vi "Dashboard Main.vi"() -> ()   [LabVIEW 2015]
uses:
  <vilib>/Utility/miscctls.llb/LVRowAndColumnTypeDef.ctl
  <vilib>/event_ctls.llb/eventvkey.ctl
  <vilib>/Rock Robotics/WPI/Dashboard/WPI_DashboardLogging Global.vi
  <vilib>/Rock Robotics/Network Tables/NT Read Numeric Array.vi
  <vilib>/Utility/config.llb/Write Key (String).vi
  <vilib>/Utility/config.llb/Write Key (I32).vi
  <vilib>/Utility/config.llb/NI_LVConfig.lvlib
panel:
  in  "TCP":refnum<k5>
  in  "Rec Mode":enum32{"Stop", "Record", "Playback"}(radio)
  in  "Vision":u16(ring) items=["Camera Off", "USB Camera SW", "USB Camera HW", "IP Camera"]
  out "Camera IP":string
  out "Image Message":string="Timeout in Camera Communications"
  in  "Dashboard Tab":T1(tab)
  in  "Select Auto":string(combo)
  out "NT Connection":bool
  in  "Camera Settings":T2={"Frame Rate"=30, "Compression"=30, "Size"=1} {"Frame Rate" scale=1.0..30.0; "Size" items=["640x480", "320x240", "160x120"]}
  out "MotorChart R":cluster{"Numeric":dbl, "Numeric":dbl}(graph)
  out "MotorChart L":T3(graph)
  out "MotorSliders R":cluster{"MotorSlide1":dbl, "MotorSlide2":dbl} {"MotorSlide2" scale=-1.0..1.0 scale format="%#_2e"; "MotorSlide1" scale=-1.0..1.0 scale format="%#_2e"}
  out "MotorSliders L":T4 {"MotorSlide4 2" scale=0.0..14.0 scale format="%#_2e"; "MotorSlide2" scale=-1.0..1.0 scale format="%#_2e"; "MotorSlide1" scale=-1.0..1.0 scale format="%#_2e"}
  out "Gyro":dbl(knob) scale=0.0..360.0
  out "JS1 Z":dbl(slide) scale=-1.0..1.0 scale format="%#_2e"
  out "JS1 Graph":cluster{"X":dbl, "Y":dbl}[](graph)
  out "JS1 Buttons":T5
  out "JS2 Z":dbl(slide) scale=-1.0..1.0 scale format="%#_2e"
  out "JS2 Graph":cluster{"X":dbl, "Y":dbl}[](graph)
  out "JS2 Buttons":T5
  out "Mode":T6(ring)=enum."Auto Disabled"
  in  "DB Camera Config":bool
  out "fps":dbl format="%#.1g"
  out "Mbps":dbl format="%#.1g"
  out "Mbps LED":bool
  in  "DB/String 9":string
  in  "DB/String 8":string
  in  "DB/String 7":string
  in  "DB/String 6":string
  in  "DB/String 5":string
  in  "DB/String 4":string
  in  "DB/String 3":string
  in  "DB/String 2":string
  in  "DB/String 1":string
  in  "DB/String 0":string
  in  "DB/Slider 0":dbl(slide) scale=0.0..5.0
  in  "DB/Slider 1":dbl(slide) scale=0.0..5.0
  in  "DB/Slider 2":dbl(slide) scale=0.0..5.0
  in  "DB/Slider 3":dbl(slide) scale=0.0..5.0
  out "DB/LED 3":bool
  out "DB/LED 2":bool
  out "DB/LED 1":bool
  out "DB/LED 0":bool
  in  "DB/Button 3":bool
  in  "DB/Button 2":bool
  in  "DB/Button 1":bool
  in  "DB/Button 0":bool caption="New Name"
  out "Velocity":dbl(knob) scale=0.0..10.0
  in  "Test Slider":dbl(slide) scale=0.0..100.0 scale format="%#_3g"
  in  "On/Off":bool caption="Solenoid"
  in  "Test Name":u16(ring) items=["Select the test to run..."]
  in  "Test Tree":string(tree)
  in  "Motor":cluster{"Value":dbl, "Enable":bool} {"Value" scale=-1.0..1.0 scale format="%#_3g"}
  out "Progress":T7 {"Test Progress" scale=0.0..100.0}
  in  "Rev/Fwd":cluster{"Forward":bool, "Reverse":bool}
  in  "Test Ring":u16(ring) items=["Monochrome", "Color"]
  out "Cmd Status":string
  in  "Execute Command":bool
  in  "Command Params":string[][](table)
  in  "Command Selection":i32(listbox)
  in  "CheckList":i32(listbox)
  out "Tree":string(tree)
  out "Camera Image":T8(plugin-control)
  out "Background":bool
  # "Left"
  # "Front"
  # "Right"
  # "Battery"
  # "This tab is a great place for autonomous settings and robot-specific values.\nPlace controls and indicators inside this tab and match name to\nDashboard Variables on robot. You can also delete this comment."
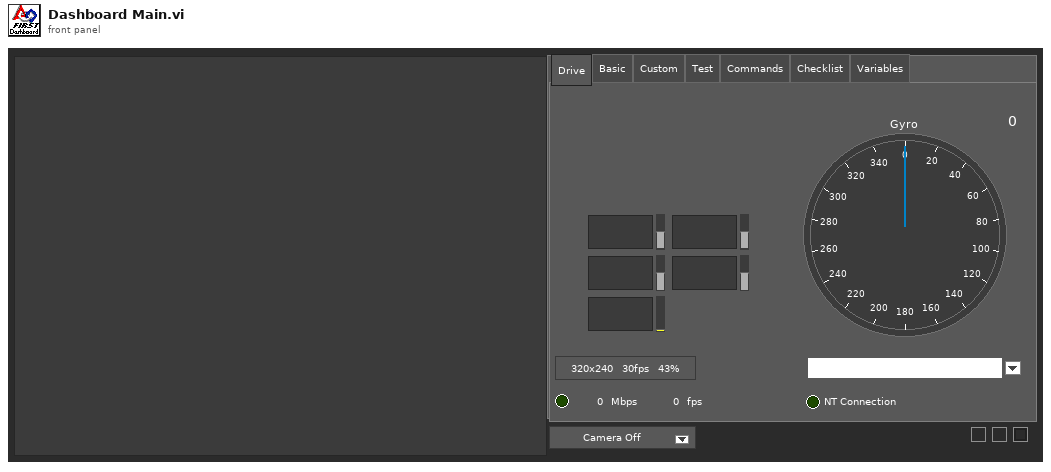
[diagram p1: front panel]
types:
  T1 = enum32{"Drive", "Basic", "Custom", "Test", "Commands", "Checklist", "Variables"}
  T2 = cluster{"Frame Rate":i32, "Compression":i32, "Size":u16}
  T3 = cluster{"Numeric":dbl, "Numeric":dbl, "Battery V":dbl}
  T4 = cluster{"MotorSlide1":dbl, "MotorSlide2":dbl, "MotorSlide4 2":dbl}
  T5 = cluster{bool, bool, bool, bool, bool, bool, bool, bool, bool, bool, bool, bool}
  T6 = enum8{"Tele-Op Disabled", "Tele-Op Enabled", "Auto Disabled", "Auto Enabled", "Test Disabled", "Test Enabled", "Disconnected", "No Code", "E-Stop"}
  T7 = cluster{"Test Progress":u8, "Test Progress Text":string}
  T8 = typedef "IMAQ Image.ctl" = refnum<image>
  T9 = cluster{"IDs":cluster{"RPC field ID":u16, "Unique ID":u16}, "String":string}
  T10 = enum32{"Drive", "Basic", "Custom", "Test", "Checklist", "Variables"}
  T11 = typedef "Image Type" = u32
  T12 = cluster{"Camera Image":refnum<vi>, "Dashboard Tab":refnum<vi>, "Background":refnum<vi>, "Vision":refnum<vi>, "Rec Mode":refnum<vi>, "Test Slider":refnum<vi>, "On/Off ":refnum<vi>, "Test Ring":refnum<vi>, "Rev/Fwd":refnum<vi>, "Test Name":refnum<vi>, "Motor":refnum<vi>, "Progress":refnum<vi>, "CheckList":refnum<vi>, "Tree":refnum<vi>, "Test Tree":refnum<vi>, "Command Params":refnum<vi>, "Command Selection":refnum<vi>, "Execute Command":refnum<vi>, "Cmd Status":refnum<vi>}
  T13 = cluster{"Error Strings":string, "Disable Counts":cluster{u16, u16}, "Rail Faults":cluster{u16, u16, u16}, "Robot IP":string, "DB Mode":u8, "Event Info":cluster{"Name":string, "Type":u8, "Number":u16, "Replay":u8}, "Camera Addr":string}
  T14 = cluster{"Storage":cluster{"Disk Free":u64, "RAM Block":u32, "RAM free":u32}, "CPU Utilization":cluster{"CPU % ISR":sgl, "CPU % Time Crit":sgl, "CPU % Timed Str":sgl, "CPU % High":sgl, "CPU % Above":sgl, "CPU % Normal":sgl, "CPU % Low":sgl}, "CAN":cluster{"% Bus Utilization":sgl, "Bus Off Cnt":u32, "TX_FIFO Full Cnt":u32, "Receive Error Cnt":u8, "Transmit Error Cnt":u8}, "HID":cluster{"HID Outputs":u32, "Rumble Low":u16, "Rumble High":u16}[]}
  T15 = cluster{"Status bits":cluster{"Test Mode":bool, "Autonomous":bool, "Enabled":bool, "Code Start":bool, "Brownout":bool, "Reserved 2":bool, "Reserved 3":bool, "E-Stop":bool}, "Code Trace":cluster{"Disabled":bool, "TeleOp":bool, "Auto":bool, "Test":bool}, "Controller Type":enum16{"unknown", "cRIO", "roboRio"}, "Code?":enum16{"unknown", "noCode", "code"}, "Battery V":dbl}
  T16 = cluster{"Control Bits":cluster{"TestMode":bool, "Autonomous":bool, "Enabled":bool, "FMS Present":bool, bool, bool, bool, "E-Stop":bool}, "Team Station ":u8, "Countdown":sgl, "Joystick Values":cluster{"Axes":dbl[], "Buttons":bool[], "POVs":i16[]}[]}
  T17 = cluster{"Axes":dbl[], "Buttons":bool[], "POVs":i16[]}[]
  T18 = cluster{"Axes":dbl[], "Buttons":bool[], "POVs":i16[]}
  T19 = cluster{"Buttons[0]":bool, "Buttons[1]":bool, "Buttons[2]":bool, "Buttons[3]":bool, "Buttons[4]":bool, "Buttons[5]":bool, "Buttons[6]":bool, "Buttons[7]":bool, "Buttons[8]":bool, "Buttons[9]":bool, "Buttons[10]":bool, "Buttons[11]":bool}
  T20 = typedef "NI_LVConfig.lvlib/Config Data RefNum.ctl" = refnum<k1>
  T21 = cluster{"Operation":enum16{"Update", "Clear"}, "Color Box":u32}[]
  T22 = typedef "eventvkey.ctl" = enum16{"ASCII", "Enter", "Return", "Shift", "Ctrl", "Alt", "Cmd", "Opt", "Caps", "NumLock", "Clear", "Break", "Up", "Down", "Left", "Right", "Insert", "Delete", "Home", "End", "PageUp", "PageDown", "Escape", "Help", "Pause", "ScrollLock", "F1", "F2", "F3", "F4", "F5", "F6", "F7", "F8", "F9", "F10", "F11", "F12", "F13", "F14", "F15", "F16", "F17", "F18", "F19", "F20", "F21", "F22", "F23", "F24", "Play", "VolumeUp", "VolumeDown", "Mute", "Two Byte Char"}
  T23 = cluster{"Image Size":bool, "Image Type":bool, "Pixel Value":bool, "ROI Information":bool, "Zoom Factor":bool}
  T24 = enum8{"Enabled", "Disabled", "Disabled and Grayed Out"}
  T25 = cluster{"Operation":enum16{"Update", "Clear"}, "Color Box":u32}
  T26 = typedef "LVRowAndColumnTypeDef.ctl" = cluster{"Row":i32, "Column":i32}
  T27 = cluster{"Shift":bool, "Ctrl":bool, "Alt":bool, "Cmd":bool, "Opt":bool}
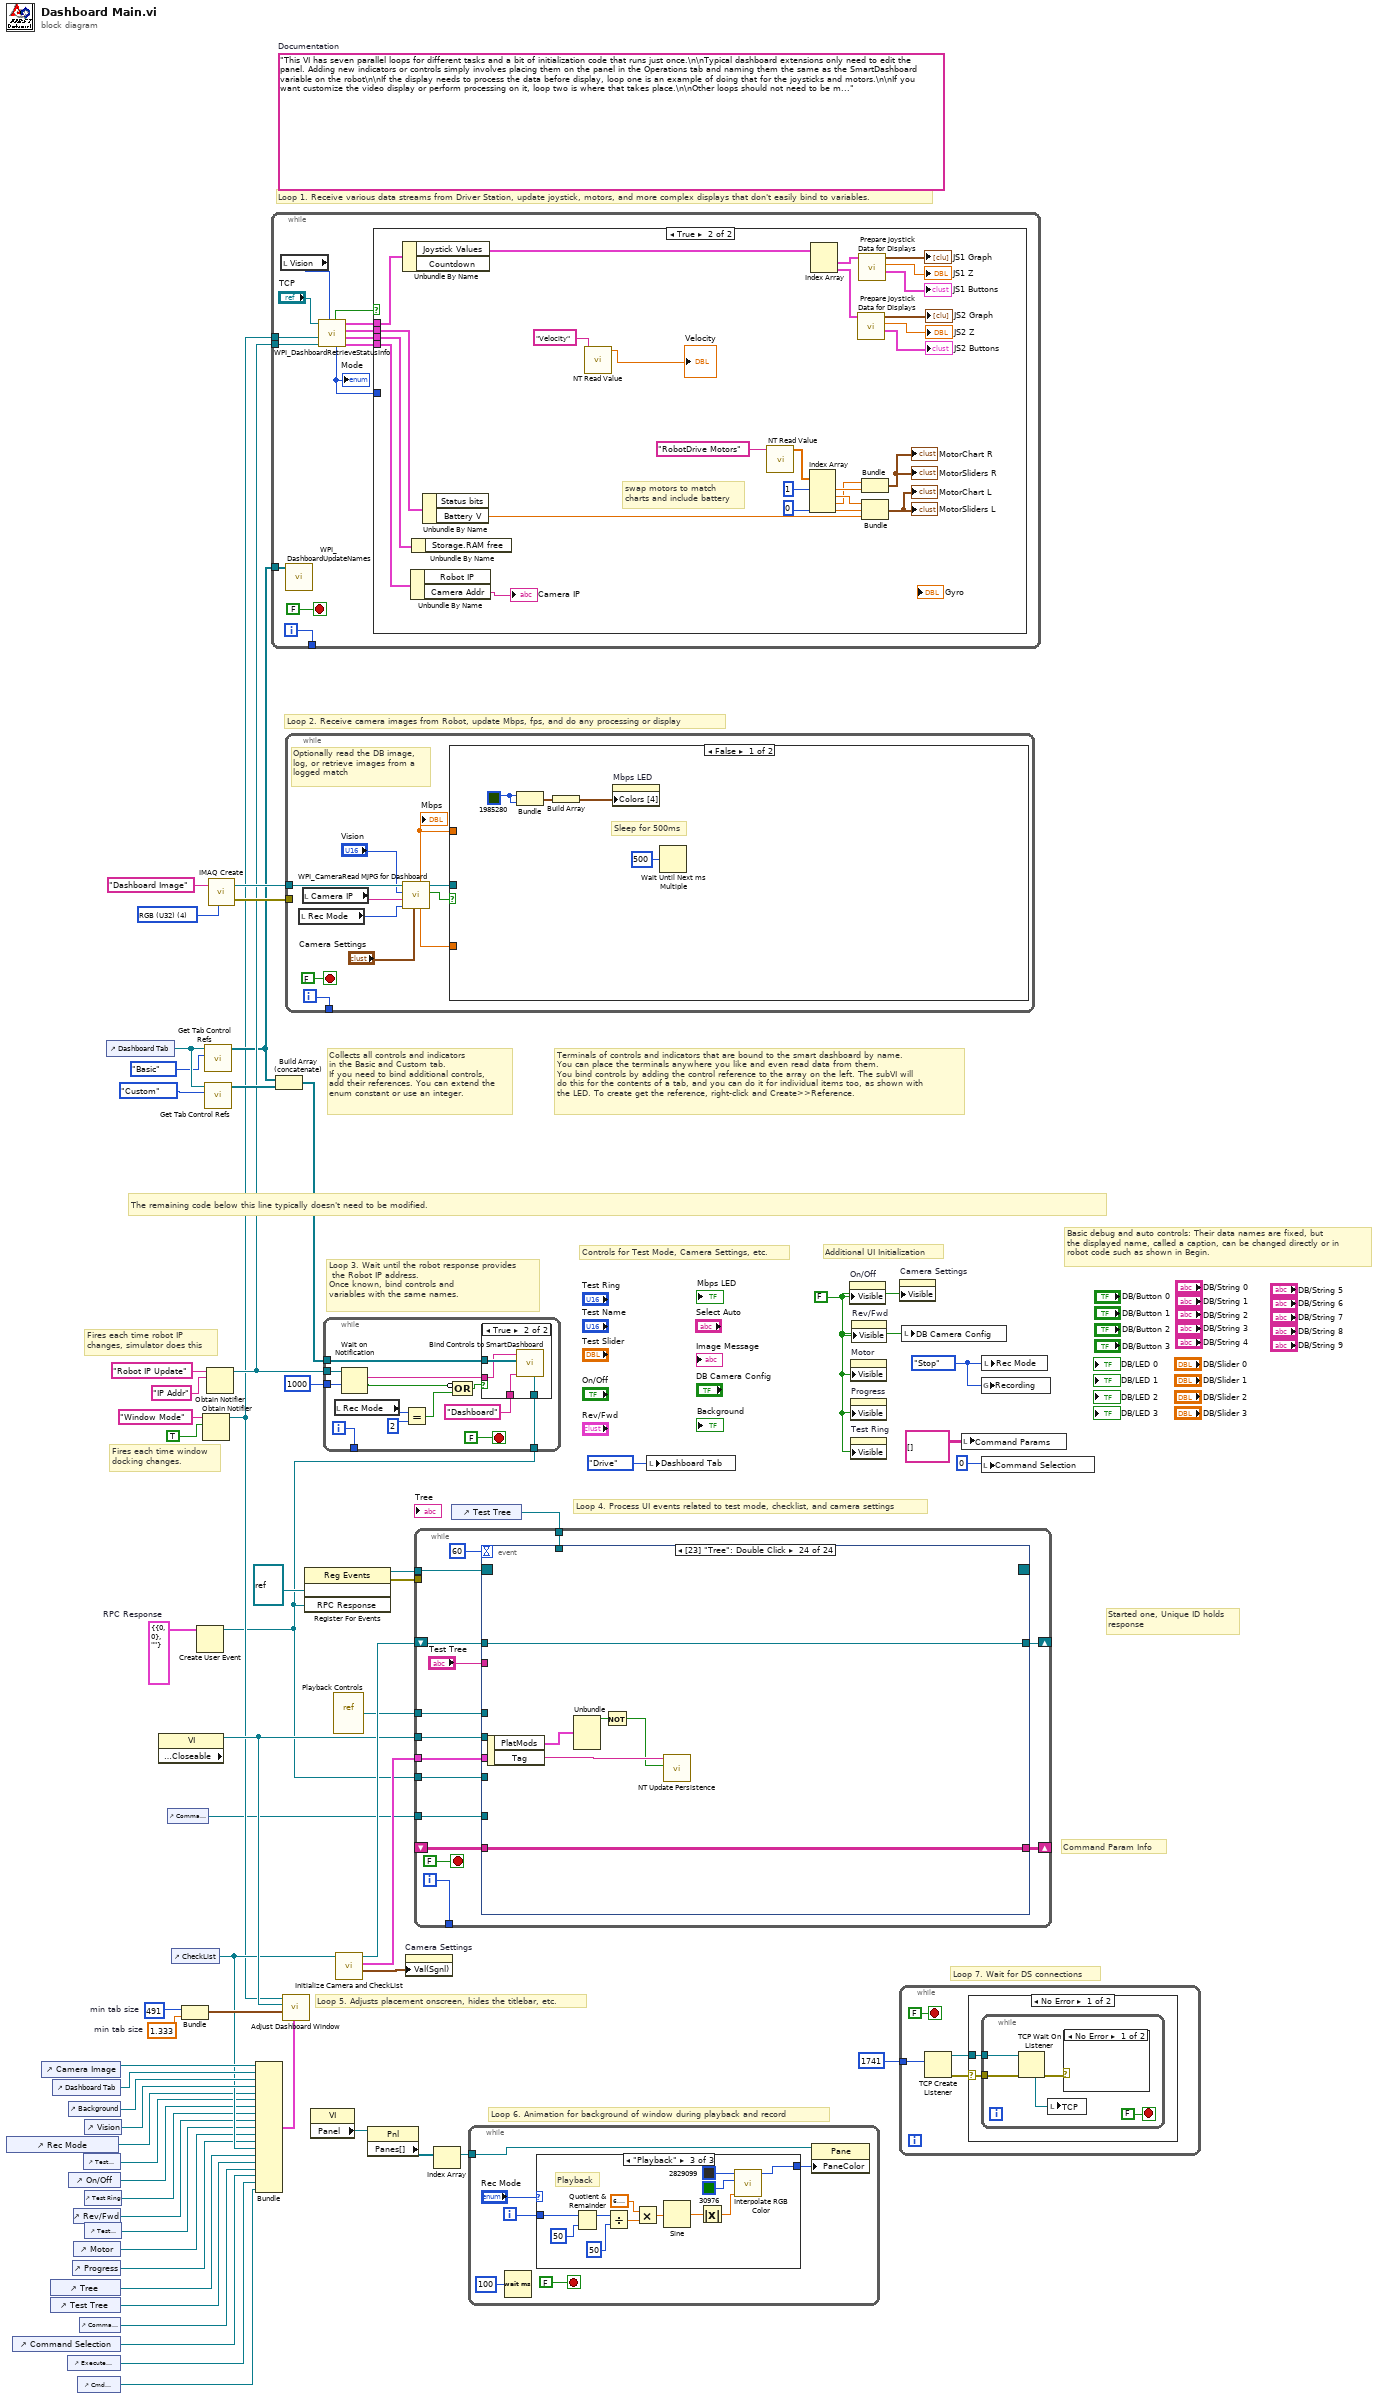
[diagram p0: block diagram]
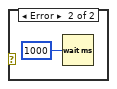
[diagram p2: hidden frame]
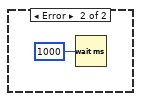
[diagram p3: hidden frame]
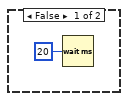
[diagram p4: hidden frame]
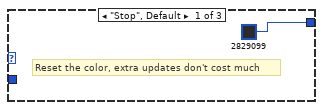
[diagram p5: hidden frame]
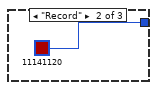
[diagram p6: hidden frame]
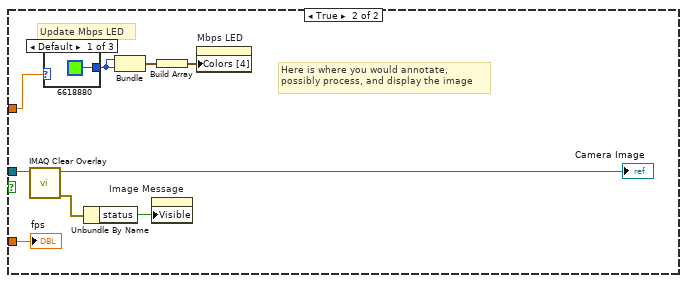
[diagram p8: hidden frame]
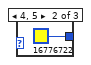
[diagram p9: hidden frame]
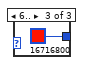
[diagram p10: hidden frame]
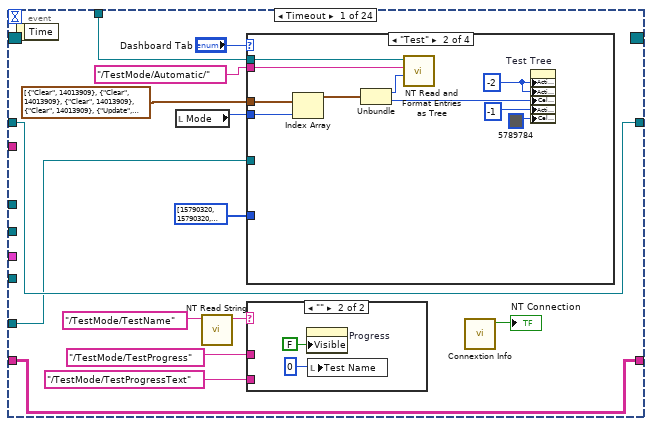
[diagram p11: hidden frame]
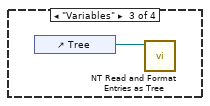
[diagram p13: hidden frame]
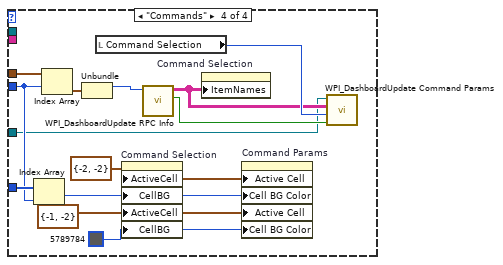
[diagram p14: hidden frame]
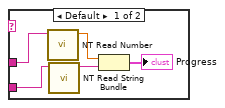
[diagram p15: hidden frame]
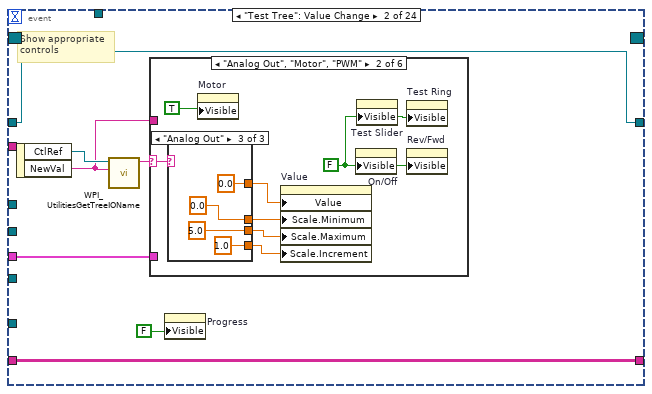
[diagram p16: hidden frame]
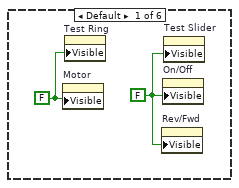
[diagram p17: hidden frame]
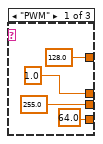
[diagram p18: hidden frame]
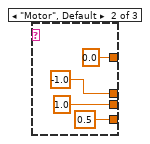
[diagram p19: hidden frame]
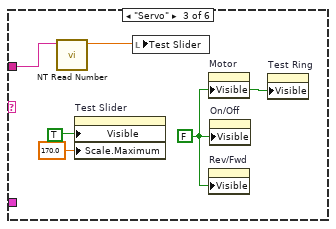
[diagram p20: hidden frame]
diagram:
  w7 = T9 {"IDs"={"RPC field ID"=0, "Unique ID"=0}, "String"=""}  # RPC Response
  w33 = 491  # min tab size
  w32 = 1.333  # min tab size
  w41 = enum32{"Stop", "Record", "Playback"}."Stop" ("Rec Mode")
  w15 = FALSE ("Visible")
  (unwired) "This VI has seven parallel loops for different tasks and a bit of initialization code that runs just once.\n\nTypical dashboard extensions only need to edit the panel. Adding new indicators or controls simply involves placing them on the panel in the Operations tab and naming them the same as the SmartDashboard variable on the robot\n\nIf the display needs to process the data before display, loop one is an example of doing that for the joysticks and motors.\n\nIf you want customize the video display or perform processing on it, loop two is where that takes place.\n\nOther loops should not need to be modified. They are pretty standard, and document the task they perform."  # Documentation
  w61 = T11 4 items=["Grayscale (U8)", "Grayscale (I16)", "Grayscale (SGL)", "Complex (CSG)", "RGB (U32)", "HSL (U32)", "RGB (U64)"] ("Image Type")
  # "Command Param Info"
  # "Started one, Unique ID holds\nresponse"
  # "Loop 7. Wait for DS connections"
  # "Basic debug and auto controls: Their data names are fixed, but\nthe displayed name, called a caption, can be changed directly or in\nrobot code such as shown in Begin."
  # "Controls for Test Mode, Camera Settings, etc."
  # "Additional UI Initialization"
  # "Loop 6. Animation for background of window during playback and record"
  # "Fires each time robot IP\nchanges, simulator does this"
  # "Fires each time window\ndocking changes."
  # "Collects all controls and indicators\nin the Basic and Custom tab.\nIf you need to bind additional controls,\nadd their references. You can extend the\nenum constant or use an integer."
  # "The remaining code below this line typically doesn't need to be modified."
  # "Loop 4. Process UI events related to test mode, checklist, and camera settings"
  # "Terminals of controls and indicators that are bound to the smart dashboard by name.\nYou can place the terminals anywhere you like and even read data from them.\nYou bind controls by adding the control reference to the array on the left. The subVI will\ndo this for the contents of a tab, and you can do it for individual items too, as shown with\nthe LED. To create get the reference, right-click and Create>>Reference."
  # "Loop 3. Wait until the robot response provides\n the Robot IP address.\nOnce known, bind controls and\nvariables with the same names."
  # "Loop 5. Adjusts placement onscreen, hides the titlebar, etc."
  # "Loop 1. Receive various data streams from Driver Station, update joystick, motors, and more complex displays that don't easily bind to variables."
  # "Loop 2. Receive camera images from Robot, update Mbps, fps, and do any processing or display"
  n1 = control-ref of="Rec Mode"() -> (w21:refnum<vi>)
  n2 = control-ref of="Command Selection"() -> (w6:refnum<vi>)
  n3 = control-ref of="Camera Image"() -> (w36:refnum<vi>)
  n4 = control-ref of="Tree"() -> (w25:refnum<vi>)
  n5 = control-ref of="Test Tree"() -> (w24:refnum<vi>)
  n6 = control-ref of="Dashboard Tab"() -> (w35:refnum<vi>)
  n7 = control-ref of="Execute Command"() -> (w8:refnum<vi>)
  n8 = control-ref of="Background"() -> (w30:refnum<vi>)
  n9 = control-ref of="On/Off"() -> (w19:refnum<vi>)
  n10 = control-ref of="Progress"() -> (w16:refnum<vi>)
  n11 = control-ref of="Rev/Fwd"() -> (w17:refnum<vi>)
  n12 = control-ref of="Motor"() -> (w22:refnum<vi>)
  n13 = control-ref of="Cmd Status"() -> (w2:refnum<vi>)
  n14 = control-ref of="Command Params"() -> (w9:refnum<vi>)
  n15 = control-ref of="Test Slider"() -> (w20:refnum<vi>)
  n16 = control-ref of="Vision"() -> (w34:refnum<vi>)
  n17 = control-ref of="Test Ring"() -> (w18:refnum<vi>)
  n18 = control-ref of="Test Name"() -> (w23:refnum<vi>)
  n19 = control-ref of="Dashboard Tab"() -> (w39:refnum<vi>)
  n20 = property class="VI" props=["Front Panel.Closeable"]() -> (reference out=w40:refnum<vi>)  [unwired: 2 in, 2 out]
  n21 = control-ref of="Command Params"() -> (w1:refnum<vi>)
  n22 = control-ref of="CheckList"() -> (w26:refnum<vi>)
  n23 = Bundle("min tab size"=w33, "min tab size"=w32) -> (w31:cluster{"min tab size":i32, "min tab size":dbl})  [unwired: 1 in]
  n24 = Create User Event(user event datatype=w7) -> (user event=w3:refnum<user-event>)  [unwired: 1 in, 1 out]
  n25 = Obtain Notifier(name (unnamed)="Window Mode", notification data type=TRUE) -> (notifier out=w12:refnum<notifier>)  [unwired: 2 in, 2 out]
  n26 = call <vilib>:"Get Tab Control Refs.vi"("Page Index"=T10."Basic" ("Dashboard Tab"), "TabControl in"=w39) -> ("ControlsOnPage"=w13:refnum<vi>[])  [unwired: 9 in]
  n27 = call <vilib>:"Get Tab Control Refs.vi"("Page Index"=T10."Custom" ("Dashboard Tab"), "TabControl in"=w39) -> ("ControlsOnPage"=w38:refnum<vi>[])  [unwired: 9 in]
  n28 = Obtain Notifier(name (unnamed)="Robot IP Update", notification data type="IP Addr" ("name (unnamed)")) -> (notifier out=w14:refnum<notifier>)  [unwired: 2 in, 2 out]
  n29 = call "IMAQ Create"("Image Name"="Dashboard Image", "Image Type"=w61) -> ("New Image"=w59:T8, "error out"=w58:errorcluster)  [unwired: 2 in, 1 out]
  n30 = Bundle("Camera Image"=w36, "Dashboard Tab"=w35, "Background"=w30, "Vision"=w34, "Rec Mode"=w21, "Test Slider"=w20, "On/Off"=w19, "Test Ring"=w18, "Rev/Fwd"=w17, "Test Name"=w23, "Motor"=w22, "Progress"=w16, "CheckList"=w26, "Tree"=w25, "Test Tree"=w24, "Command Params"=w9, "Command Selection"=w6, "Execute Command"=w8, "Cmd Status"=w2) -> (w27:T12)  [unwired: 1 in]
  n31 = while {
    tunnel: [w73] -> _
    tunnel: w14 -> [w67]
    tunnel: w13 -> [w66]
    tunnel: w12 -> [w62]
    i -> [w73]
    stop <- FALSE stop-if-true
    n32 = local read "Vision"() -> (w64:u16)
    n33 = call <vilib>:"WPI_DashboardUpdateNames.vi"("Controls on Tab"=w66) -> ()  [unwired: 11 in]
    n34 = call <vilib>:"WPI_DashboardRetrieveStatusInfo.vi"("Vision"=w64, "Binding Refnum"=w67, "Window Mode Notifier"=w62, "TCP Cnx"="TCP") -> ("Power and Errors"=w68:T13, "Robot Metrics"=w71:T14, "Status Info"=w72:T15, "Control Info"=w69:T16, "Robot Mode"=w65:T6, "Process?"=w70:bool)  [unwired: 2 in]
    "Mode" <- w65
    n35 = case shown="True" w70 {
      tunnel: w72 -> [_ w102]
      tunnel: w71 -> [_ w101]
      tunnel: w69 -> [_ w100]
      tunnel: w68 -> [_ w99]
      tunnel: w65 -> [_ _]
      frame False {
        n36 = Wait (ms)(milliseconds to wait=u32 20) -> ()  [unwired: 1 out]
      }
      frame True {
        # "swap motors to match\ncharts and include battery"
        n37 = Unbundle By Name(w100) -> ("Joystick Values"=w89:T17)  [unwired: 1 out]
        n38 = Unbundle By Name(w99) -> ("Camera Addr"=→"Camera IP":string)  [unwired: 1 out]
        n39 = Unbundle By Name(w101) -> ()  [unwired: 1 out]
        n40 = Unbundle By Name(w102) -> ("Battery V"=w90:dbl)  [unwired: 1 out]
        n41 = call-poly <vilib>:"NT Read Value.vi"("Name"="Velocity") -> ("Numeric"=→"Velocity":dbl)  [unwired: 9 in, 1 out]
        n42 = call-poly <vilib>:"NT Read Value.vi"("Name"="RobotDrive Motors") -> ("Numeric Array"=w78:dbl[])  [unwired: 9 in, 1 out]
        n43 = Index Array(array=w78, index #1=1, index #4=0) -> (element #1=w94:dbl, element #2=w95:dbl, element #3=w93:dbl, element #4=w98:dbl)  [unwired: 2 in]
        n44 = Index Array(array=w89) -> (element #1=w88:T18, element #2=w83:T18)  [unwired: 2 in]
        n45 = call "Prepare Joystick Data for Displays.vi"("Joystick Values"=w83) -> ("Buttons"=→"JS2 Buttons":T19, "Z Axis"=→"JS2 Z":dbl, "Cartesian Data"=→"JS2 Graph":cluster{"X axis":dbl, "X axis":dbl}[])  [unwired: 8 in]
        n46 = call "Prepare Joystick Data for Displays.vi"("Joystick Values"=w88) -> ("Buttons"=→"JS1 Buttons":T19, "Z Axis"=→"JS1 Z":dbl, "Cartesian Data"=→"JS1 Graph":cluster{"X axis":dbl, "X axis":dbl}[])  [unwired: 8 in]
        n47 = Bundle("Numeric"=w93, "Numeric"=w94) -> (→"MotorChart R" →"MotorSliders R":cluster{"Numeric":dbl, "Numeric":dbl})  [unwired: 1 in]
        n48 = Bundle("Numeric"=w95, "Numeric"=w98, "Battery V"=w90) -> (→"MotorChart L" →"MotorSliders L":T3)  [unwired: 1 in]
      }
    }
  }
  n49 = Build Array (concatenate)(w13, w38) -> (w37:refnum<vi>[])
  n50 = call "Adjust Dashboard Window.vi"("Sizing Refnums"=w27, "Size Constraints"=w31, "VI"=w40, "WIn Mode"=w12) -> ()  [unwired: 8 in]
  n51 = while {
    tunnel: w59 -> [w111]
    tunnel: w58 -> [_]
    tunnel: [w112] -> _
    i -> [w112]
    stop <- FALSE stop-if-true
    # "Optionally read the DB image,\nlog, or retrieve images from a\nlogged match"
    n52 = local read "Rec Mode"() -> (w106:enum32{"Stop", "Record", "Playback"})
    n53 = local read "Camera IP"() -> (w104:string)
    n54 = call <vilib>:"WPI_CameraRead MJPG for Dashboard.vi"("Camera Settings"="Camera Settings", "Rec Mode"=w106, "Camera IP"=w104, "Camera Mode"="Vision", "Refnum in"=w111) -> ("Active"=w109:bool, "Refnum out"=w110:T8, "FPS"=w108:dbl, "Bandwidth (Mbps)"=w103:dbl)  [unwired: 3 in]
    "Mbps" <- w103
    n55 = case shown="False" w109 {
      tunnel: w110 -> [_ w121]
      tunnel: w103 -> [_ w120]
      tunnel: w108 -> [_ w118]
      frame False {
        w114 = u32 1985280 ("Color Box")
        # "Sleep for 500ms"
        n56 = Bundle("Color Box"=w114, "Color Box"=w114) -> (w116:cluster{"Color Box":u32, "Color Box":u32})  [unwired: 1 out]
        n57 = Build Array(w116) -> (w115:cluster{"Color Box":u32, "Color Box":u32}[])
        n58 = property on="Mbps LED" class="Bool (strict)"("Colors [4]"=w115) -> ()  [unwired: 2 in, 2 out]
        n59 = Wait Until Next ms Multiple(millisecond multiple=u32 500) -> ()  [unwired: 1 out]
      }
      frame True {
        # "Here is where you would annotate,\npossibly process, and display the image"
        # "Update Mbps LED"
        n60 = call "IMAQ Clear Overlay"("Image"=w121) -> ("error out"=w125:errorcluster, "Image Out"=→"Camera Image":T8)  [unwired: 2 in, 7 out]
        n61 = case shown="Default" w120 {
          tunnel: [u32 6618880 ("Color Box") u32 16776722 ("Color Box") u32 16716800 ("Color Box")] -> w122
          frame Default {
          }
          frame 4, 5 {
          }
          frame 6.. {
          }
        }
        n62 = Unbundle By Name(w125) -> ("status"=w126:bool)
        n63 = Bundle("Color Box"=w122, "Color Box"=w122) -> (w124:cluster{"Color Box":u32, "Color Box":u32})  [unwired: 1 out]
        n64 = property on="Image Message" class="Str"("Visible"=w126) -> ()  [unwired: 2 in, 2 out]
        n65 = Build Array(w124) -> (w123:cluster{"Color Box":u32, "Color Box":u32}[])
        n66 = property on="Mbps LED" class="Bool (strict)"("Colors [4]"=w123) -> ()  [unwired: 2 in, 2 out]
        "fps" <- w118
      }
    }
  }
  n67 = register-events(refnum<vi> refnum, w3) -> (reference out=w45:refnum<event-registration>, error out=w44:errorcluster)  [unwired: 2 in]
  n68 = property class="VI"() -> ("Panel"=w48:refnum<vi>)  [unwired: 2 in, 2 out]
  n69 = while {
    tunnel: w37 -> [w142]
    tunnel: w14 -> [w140]
    tunnel: [w138] -> _
    tunnel: u32 1000 ("milliseconds to wait") -> [w137]
    tunnel: w3 -> [w130]
    i -> [w138]
    stop <- FALSE stop-if-true
    n70 = local read "Rec Mode"() -> (w133:enum32{"Stop", "Record", "Playback"})
    n71 = Wait on Notification(notifier=w140, timeout in ms (-1)=w137) -> (notification=w139:string, timed out?=w135:bool)  [unwired: 2 in, 2 out]
    n72 = Equal?(x=w133, y=u16 2 ("Rec Mode")) -> (x = y?=w134:bool)
    n73 = Compound Arithmetic op=OR(invert w135, w134) -> (w136:bool)
    n74 = case shown="True" w136 {
      tunnel: w142 -> [_ w146]
      tunnel: w139 -> [_ w145]
      tunnel: "Dashboard" -> [_ w144]
      tunnel: w130 -> [_ w143]
      frame False {
      }
      frame True {
        n75 = call <vilib>:"Bind Controls to SmartDashboard.vi"("RPC ref"=w143, "Client Name"=w144, "Bound Control Refs"=w146, "Server IP Address"=w145) -> ()  [unwired: 8 in]
      }
    }
  }
  n76 = vi-ref "Playback Controls.vi"() -> (w46:refnum<vi>)
  n77 = call "Initialize Camera and CheckList.vi"("ListBox in"=w26) -> ("Cluster"=w52:cluster{"value":i32, "value":i32, "index":i32}, "Array"=w53:cluster{string[]}[], "File Refnum"=w51:T20)  [unwired: 8 in]
  n78 = property class="Pnl"(reference=w48) -> ("Panes[]"=w49:refnum<vi>[])  [unwired: 1 in, 2 out]
  n79 = property on="Camera Settings" class="Clust (strict)"("Val(Sgnl)"=w52) -> ()  [unwired: 2 in, 2 out]
  n80 = Index Array(array=w49) -> (element=w47:refnum<vi>)  [unwired: 1 in]
  n81 = control-ref of="Test Tree"() -> (w50:refnum<vi>)
  n82 = while {
    tunnel: w53 -> [w158]
    shift-right: [w157] -> _
    shift-left: w51 -> [w156]
    tunnel: [w155] -> _
    tunnel: w50 -> [w154]
    tunnel: w46 -> [w153]
    tunnel: w45 -> [w152]
    tunnel: w44 -> [_]
    tunnel: w40 -> [w151]
    tunnel: w3 -> [w150]
    tunnel: w1 -> [w149]
    shift-right: [w148] -> _
    shift-left: _ -> [w147]
    i -> [w155]
    stop <- FALSE stop-if-true
    n83 = event shown="[23] \"Tree\": Double Click" {
      selector: w152 -> [_ _ _ _ _ _ _ _ _ _ _ _ _ _ _ _ _ _ _ _ _ _ _ _]
      dyn-events: [_ _ _ _ _ _ _ _ _ _ _ _ _ _ _ _ _ _ w467 _ _ _ _ _] -> _
      timeout: u32 60 ("milliseconds to wait") -> [_ _ _ _ _ _ _ _ _ _ _ _ _ _ _ _ _ _ _ _ _ _ _ _]
      tunnel: w154 -> [w171 _ _ _ _ _ _ _ _ _ _ _ _ _ _ _ _ _ _ _ _ _ _ _]
      tunnel: "Test Tree" -> [_ _ _ _ _ _ _ _ _ _ _ _ _ w430 w439 w442 w447 w456 _ _ _ _ _ _]
      tunnel: w158 -> [_ w209 _ _ _ _ _ _ _ _ _ w392 w423 _ _ _ _ _ _ _ _ _ _ _]
      tunnel: [w168 w208 w312 w318 w328 w332 w338 w350 w358 w364 w377 w391 w416 w429 w437 w441 w446 w455 w469 w485 w487 w495 w506 w511] -> w157
      tunnel: w156 -> [w168 w208 w312 w318 w328 w332 w338 w350 w358 w364 w377 w390 w416 w429 w437 w441 w446 w455 w469 w485 w487 w495 w506 w511]
      tunnel: w153 -> [_ _ _ _ _ _ _ _ _ _ _ _ _ _ _ _ _ _ w470 _ w490 _ _ _]
      tunnel: w151 -> [_ _ _ _ _ _ _ _ _ _ _ _ _ _ _ _ _ _ w465 _ _ _ _ _]
      tunnel: w150 -> [_ _ _ _ _ _ _ _ _ _ _ _ _ _ _ _ _ _ w461 _ _ _ _ _]
      tunnel: w149 -> [w163 _ _ _ _ _ w336 _ _ _ _ _ _ _ _ _ _ _ _ _ _ _ _ _]
      tunnel: [w162 w207 w311 w317 w327 w333 w334 w344 w355 w363 w376 w389 w415 w428 w436 w440 w445 w454 w460 w483 w486 w491 w499 w512] -> w148
      tunnel: w147 -> [w162 w207 w311 w317 w327 w333 w334 _ _ w363 w376 w389 w415 w428 w436 w440 w445 w454 w460 w483 w486 w491 w499 w512]
      event Timeout {
        n84 = event-data() -> ()  [unwired: 1 in, 1 out]
        n85 = local read "Mode"() -> (w165:T6)
        n86 = call <vilib>:"NT Read String.vi"("Name"="/TestMode/TestName") -> ("String"=w174:string)  [unwired: 9 in, 1 out]
        n87 = case shown="\"Test\"" "Dashboard Tab" {
          tunnel: w171 -> [_ w185 _ _]
          tunnel: "/TestMode/Automatic/" ("Name Pattern") -> [_ w184 _ _]
          tunnel: T21 [{"Operation"=enum."Clear", "Color Box"=14013909}, {"Operation"=enum."Clear", "Color Box"=14013909}, {"Operation"=enum."Clear", "Color Box"=14013909}, {"Operation"=enum."Clear", "Color Box"=14013909}, {"Operation"=enum."Update", "Color Box"=14013909}, {"Operation"=enum."Update", "Color Box"=16777215}, {"Operation"=enum."Clear", "Color Box"=14013909}, {"Operation"=enum."Clear", "Color Box"=14013909}, {"Operation"=enum."Clear", "Color Box"=14013909}] -> [_ w177 _ w194]
          tunnel: w165 -> [_ w176 _ w193]
          tunnel: u32[] [15790320, 15790320, 15790320, 15790320, 16777215, 16777215, 15790320, 15790320, 15790320] -> [_ _ _ w199]
          tunnel: w163 -> [_ _ _ w187]
          frame "Custom", Default {
          }
          frame "Test" {
            w183 = -2 ("Active Item:Row Number")
            n88 = Index Array(array=w177, index=w176) -> (element=w178:T25)
            n89 = Unbundle(w178) -> ("Operation"=w179:enum16{"Update", "Clear"}, "Color Box"=w180:u32)
            n90 = call <vilib>:"NT Read and Format Entries as Tree.vi"("Operation"=w179, "Name Pattern"=w184, "Tree Refnum"=w185) -> ()  [unwired: 7 in, 2 out]
            n91 = property on="Test Tree" class="Tree (strict)"("Active Item Row Number"=w183, "ActiveColNum"=w183, "CellBG"=w180, "Active Item Row Number"=-1 ("Active Item:Row Number"), "CellBG"=u32 5789784 ("Color Box")) -> ()  [unwired: 2 in, 2 out]
          }
          frame "Variables" {
            n92 = control-ref of="Tree"() -> (w186:refnum<vi>)
            n93 = call <vilib>:"NT Read and Format Entries as Tree.vi"("Tree Refnum"=w186) -> ()  [unwired: 9 in, 2 out]
          }
          frame "Commands" {
            w195 = u32 5789784 ("Color Box")
            w196 = T26 {"Row"=-1, "Column"=-2} ("Active Cell:Active Cell")
            w198 = T26 {"Row"=-2, "Column"=-2} ("Active Cell:Active Cell")
            n94 = Index Array(array=w199, index=w193) -> (element=w197:u32)
            n95 = Index Array(array=w194, index=w193) -> (element=w192:T25)
            n96 = Unbundle(w192) -> ("Operation"=w191:enum16{"Update", "Clear"})  [unwired: 1 out]
            n97 = local read "Command Selection"() -> (w190:i32)
            n98 = property on="Command Selection" class="MCListbox (strict)"("ActiveCell"=w198, "CellBG"=w197, "ActiveCell"=w196, "CellBG"=w195) -> ()  [unwired: 2 in, 2 out]
            n99 = call <vilib>:"WPI_DashboardUpdate RPC Info.vi"("Operation"=w191) -> ("update"=w189:bool, "commands"=w188:string[][])  [unwired: 9 in]
            n100 = property on="Command Selection" class="MCListbox (strict)"("ItemNames"=w188) -> ()  [unwired: 2 in, 2 out]
            n101 = property on="Command Params" class="Tbl (strict)"("Active Cell"=w198, "Cell BG Color"=w197, "Active Cell"=w196, "Cell BG Color"=w195) -> ()  [unwired: 2 in, 2 out]
            n102 = call <vilib>:"WPI_DashboardUpdate Command Params.vi"("Update"=w189, "NewVal"=w190, "Commands"=w188, "Param Tbl"=w187) -> ()  [unwired: 7 in, 1 out]
          }
        }
        n103 = case shown="\"\"" w174 {
          tunnel: "/TestMode/TestProgress" ("Name") -> [w201 _]
          tunnel: "/TestMode/TestProgressText" ("Name") -> [w200 _]
          frame Default {
            n104 = call <vilib>:"NT Read Number.vi"("Name"=w201) -> ("Numeric"=w202:dbl)  [unwired: 9 in, 1 out]
            n105 = call <vilib>:"NT Read String.vi"("Name"=w200) -> ("String"=w203:string)  [unwired: 9 in, 1 out]
            n106 = Bundle("Numeric"=w202, "String"=w203) -> (→"Progress":cluster{"Numeric":dbl, "String":string})  [unwired: 1 in]
          }
          frame "" {
            n107 = property on="Progress" class="Clust (strict)"("Visible"=FALSE) -> ()  [unwired: 2 in, 2 out]
            n108 = local write "Test Name"(u16 0) -> ()
          }
        }
        n109 = call <vilib>:"Connextion Info.vi"() -> ("Connected"=→"NT Connection":bool)  [unwired: 10 in, 1 out]
      }
      event "Test Tree": Value Change {
        # "Show appropriate\ncontrols"
        n110 = event-data() -> ("CtlRef"=w212:refnum<vi>, "NewVal"=w210:string)  [unwired: 1 in]
        n111 = call <vilib>:"WPI_UtilitiesGetTreeIOName.vi"("NewVal"=w210, "TreeControl in"=w212) -> ("I/O Name"=w213:string)  [unwired: 9 in]
        n112 = case shown="\"Analog Out\", \"Motor\", \"PWM\"" w213 {
          selector: w213 -> [_ w220 _ w242 w251 _]
          tunnel: w210 -> [_ _ w239 w241 _ w258]
          tunnel: w209 -> [_ _ _ _ _ w257]
          frame Default {
            w215 = FALSE ("Visible")
            w214 = FALSE ("Visible")
            n113 = property on="Motor" class="Clust (strict)"("Visible"=w214) -> ()  [unwired: 2 in, 2 out]
            n114 = property on="Test Ring" class="Ring (strict)"("Visible"=w214) -> ()  [unwired: 2 in, 2 out]
            n115 = property on="Rev/Fwd" class="Clust (strict)"("Visible"=w215) -> ()  [unwired: 2 in, 2 out]
            n116 = property on="On/Off" class="Bool (strict)"("Visible"=w215) -> ()  [unwired: 2 in, 2 out]
            n117 = property on="Test Slider" class="Slide (strict)"("Visible"=w215) -> ()  [unwired: 2 in, 2 out]
          }
          frame "Analog Out", "Motor", "PWM" {
            w221 = FALSE ("Visible")
            n118 = case shown="\"Analog Out\"" w220 {
              tunnel: [1.0 ("Value") -1.0 ("Value") 0.0 ("Value")] -> w219
              tunnel: [255.0 ("Value") 1.0 ("Value") 5.0 ("Value")] -> w218
              tunnel: [128.0 ("Value") 0.0 ("Value") 0.0 ("Value")] -> w217
              tunnel: [64.0 ("Value") 0.5 ("Value") 1.0 ("Value")] -> w216
              frame "PWM" {
              }
              frame "Motor", Default {
              }
              frame "Analog Out" {
              }
            }
            n119 = property on="Motor" class="Clust (strict)"("Visible"=TRUE) -> ()  [unwired: 2 in, 2 out]
            n120 = property on="Value" class="Slide (strict)"("Value"=w217, "Scale.Minimum"=w219, "Scale.Maximum"=w218, "Scale.Increment"=w216) -> ()  [unwired: 2 in, 2 out]
            n121 = property on="On/Off" class="Bool (strict)"("Visible"=w221) -> ()  [unwired: 2 in, 2 out]
            n122 = property on="Test Slider" class="Slide (strict)"("Visible"=w221) -> ()  [unwired: 2 in, 2 out]
            n123 = property on="Test Ring" class="Ring (strict)"("Visible"=w221) -> ()  [unwired: 2 in, 2 out]
            n124 = property on="Rev/Fwd" class="Clust (strict)"("Visible"=w221) -> ()  [unwired: 2 in, 2 out]
          }
          frame "Servo" {
            w237 = FALSE ("Visible")
            n125 = call <vilib>:"NT Read Number.vi"("Name"=w239) -> ("Numeric"=w238:dbl)  [unwired: 9 in, 1 out]
            n126 = property on="Test Slider" class="Slide (strict)"("Visible"=TRUE, "Scale.Maximum"=170.0 ("Scale.Range:Maximum")) -> ()  [unwired: 2 in, 2 out]
            n127 = local write "Test Slider"(w238) -> ()
            n128 = property on="Motor" class="Clust (strict)"("Visible"=w237) -> ()  [unwired: 2 in, 2 out]
            n129 = property on="Rev/Fwd" class="Clust (strict)"("Visible"=w237) -> ()  [unwired: 2 in, 2 out]
            n130 = property on="On/Off" class="Bool (strict)"("Visible"=w237) -> ()  [unwired: 2 in, 2 out]
            n131 = property on="Test Ring" class="Ring (strict)"("Visible"=w237) -> ()  [unwired: 2 in, 2 out]
          }
          frame "Relay", "Solenoid" {
            w240 = FALSE ("Visible")
            n132 = property on="Motor" class="Clust (strict)"("Visible"=w240) -> ()  [unwired: 2 in, 2 out]
            n133 = property on="Test Slider" class="Slide (strict)"("Visible"=w240) -> ()  [unwired: 2 in, 2 out]
            n134 = Search and Replace String(input string=w241, search string="/Value  **", replace string="/Direction") -> (result string=w247:string)  [unwired: 5 in, 3 out]
            n135 = property on="Test Ring" class="Ring (strict)"("Visible"=w240) -> ()  [unwired: 2 in, 2 out]
            n136 = call <vilib>:"NT Read String.vi"("Name"=w247) -> ("String"=w245:string)  [unwired: 9 in, 1 out]
            n137 = Equal?(x="Both directions", y=w245) -> (x = y?=w243:bool)
            n138 = Not(x=w243) -> (.not. x?=w244:bool)
            n139 = property on="Rev/Fwd" class="Clust (strict)"("Visible"=w243) -> ()  [unwired: 2 in, 2 out]
            n140 = property on="On/Off" class="Bool (strict)"("Visible"=w244, "Caption.Text"=w242) -> ()  [unwired: 2 in, 2 out]
          }
          frame "Compressor", "Digital Out" {
            w250 = FALSE ("Visible")
            # "Get direction and finish"
            n141 = property on="Motor" class="Clust (strict)"("Visible"=w250) -> ()  [unwired: 2 in, 2 out]
            n142 = property on="Test Slider" class="Slide (strict)"("Visible"=w250) -> ()  [unwired: 2 in, 2 out]
            n143 = property on="Test Ring" class="Ring (strict)"("Visible"=w250) -> ()  [unwired: 2 in, 2 out]
            n144 = property on="On/Off" class="Bool (strict)"("Visible"=TRUE, "Caption.Text"=w251) -> ()  [unwired: 2 in, 2 out]
            n145 = property on="Rev/Fwd" class="Clust (strict)"("Visible"=FALSE) -> ()  [unwired: 2 in, 2 out]
          }
          frame "Camera" {
            n146 = call <vilib>:"Get Last Path Segment.vi"("String in"=w258) -> ("String out"=w259:string)  [unwired: 10 in]
            n147 = property on="On/Off" class="Bool (strict)"("Visible"=FALSE) -> ()  [unwired: 2 in, 2 out]
            n148 = property on="Motor" class="Clust (strict)"("Visible"=FALSE) -> ()  [unwired: 2 in, 2 out]
            n149 = property on="Rev/Fwd" class="Clust (strict)"("Visible"=FALSE) -> ()  [unwired: 2 in, 2 out]
            n150 = case shown="\"White Balance  **\"" w259 {
              tunnel: w258 -> [w265 w274 w283 w292 w301 _ w307]
              tunnel: w257 -> [w263 w271 w280 w289 w298 _ _]
              frame "Size  **" {
                n151 = Index Array(array=w263) -> (element=w262:cluster{string[]})  [unwired: 1 in]
                n152 = call <vilib>:"NT Read String.vi"("Name"=w265) -> ("String"=w264:string)  [unwired: 9 in, 1 out]
                n153 = Unbundle(w262) -> (w260:string[])
                n154 = Match First String(2:w260, 3:w264) -> (0:w261:i32)  [unwired: 1 out]
                n155 = property on="Test Ring" class="Ring (strict)"("Value"=w261, "Strings []"=w260) -> ()  [unwired: 2 in, 2 out]
                n156 = property on="Test Ring" class="Ring (strict)"("Visible"=TRUE) -> ()  [unwired: 2 in, 2 out]
                n157 = property on="Test Slider" class="Slide (strict)"("Visible"=FALSE) -> ()  [unwired: 2 in, 2 out]
              }
              frame "White Balance  **" {
                n158 = Index Array(array=w271, index=1) -> (element=w272:cluster{string[]})
                n159 = call <vilib>:"NT Read String.vi"("Name"=w274) -> ("String"=w273:string)  [unwired: 9 in, 1 out]
                n160 = Unbundle(w272) -> (w269:string[])
                n161 = Match First String(2:w269, 3:w273) -> (0:w268:i32)  [unwired: 1 out]
                n162 = property on="Test Ring" class="Ring (strict)"("Value"=w268, "Strings []"=w269) -> ()  [unwired: 2 in, 2 out]
                n163 = property on="Test Ring" class="Ring (strict)"("Visible"=TRUE) -> ()  [unwired: 2 in, 2 out]
                n164 = property on="Test Slider" class="Slide (strict)"("Visible"=FALSE) -> ()  [unwired: 2 in, 2 out]
              }
              frame "Exposure  **" {
                n165 = Index Array(array=w280, index=2) -> (element=w281:cluster{string[]})
                n166 = call <vilib>:"NT Read String.vi"("Name"=w283) -> ("String"=w282:string)  [unwired: 9 in, 1 out]
                n167 = Unbundle(w281) -> (w277:string[])
                n168 = Match First String(2:w277, 3:w282) -> (0:w278:i32)  [unwired: 1 out]
                n169 = property on="Test Ring" class="Ring (strict)"("Value"=w278, "Strings []"=w277) -> ()  [unwired: 2 in, 2 out]
                n170 = property on="Test Ring" class="Ring (strict)"("Visible"=TRUE) -> ()  [unwired: 2 in, 2 out]
                n171 = property on="Test Slider" class="Slide (strict)"("Visible"=FALSE) -> ()  [unwired: 2 in, 2 out]
              }
              frame "Exposure Priority  **" {
                n172 = Index Array(array=w289, index=3) -> (element=w290:cluster{string[]})
                n173 = call <vilib>:"NT Read String.vi"("Name"=w292) -> ("String"=w291:string)  [unwired: 9 in, 1 out]
                n174 = Unbundle(w290) -> (w286:string[])
                n175 = Match First String(2:w286, 3:w291) -> (0:w287:i32)  [unwired: 1 out]
                n176 = property on="Test Ring" class="Ring (strict)"("Value"=w287, "Strings []"=w286) -> ()  [unwired: 2 in, 2 out]
                n177 = property on="Test Ring" class="Ring (strict)"("Visible"=TRUE) -> ()  [unwired: 2 in, 2 out]
                n178 = property on="Test Slider" class="Slide (strict)"("Visible"=FALSE) -> ()  [unwired: 2 in, 2 out]
              }
              frame "Color Enable  **" {
                n179 = Index Array(array=w298, index=4) -> (element=w299:cluster{string[]})
                n180 = call <vilib>:"NT Read String.vi"("Name"=w301) -> ("String"=w300:string)  [unwired: 9 in, 1 out]
                n181 = Unbundle(w299) -> (w295:string[])
                n182 = Match First String(2:w295, 3:w300) -> (0:w296:i32)  [unwired: 1 out]
                n183 = property on="Test Ring" class="Ring (strict)"("Value"=w296, "Strings []"=w295) -> ()  [unwired: 2 in, 2 out]
                n184 = property on="Test Ring" class="Ring (strict)"("Visible"=TRUE) -> ()  [unwired: 2 in, 2 out]
                n185 = property on="Test Slider" class="Slide (strict)"("Visible"=FALSE) -> ()  [unwired: 2 in, 2 out]
              }
              frame Default {
                n186 = property on="Test Ring" class="Ring (strict)"("Visible"=FALSE) -> ()  [unwired: 2 in, 2 out]
                n187 = property on="Test Slider" class="Slide (strict)"("Visible"=FALSE) -> ()  [unwired: 2 in, 2 out]
              }
              frame "Brightness  **", "Color Level  **", "Compression  **", "FPS  **", "Sharpness  **" {
                n188 = call <vilib>:"NT Read Number.vi"("Name"=w307) -> ("Numeric"=w306:dbl)  [unwired: 9 in, 1 out]
                n189 = local write "Test Slider"(w306) -> ()
                n190 = property on="Test Slider" class="Slide (strict)"("Visible"=TRUE, "Scale.Maximum"=100.0 ("Scale.Range:Maximum")) -> ()  [unwired: 2 in, 2 out]
                n191 = property on="Test Ring" class="Ring (strict)"("Visible"=FALSE) -> ()  [unwired: 2 in, 2 out]
              }
            }
          }
        }
        n192 = property on="Progress" class="Clust (strict)"("Visible"=FALSE) -> ()  [unwired: 2 in, 2 out]
      }
      event "Test Name": Mouse Enter {
        # "Populate the ring with the list of tests"
        n193 = event-data() -> ()  [unwired: 1 in, 1 out]
        n194 = call <vilib>:"NT Read String Array.vi"("Name"="/TestMode/TestList") -> ("String Array"=w316:string[])  [unwired: 9 in, 1 out]
        n195 = Build Array (concatenate)("Select the test to run...", w316) -> (w315:string[])
        n196 = property on="Test Name" class="Ring (strict)"("Strings []"=w315) -> ()  [unwired: 2 in, 2 out]
      }
      event "Test Name": Value Change {
        w319 = FALSE ("Visible")
        # "Tell the robot the test name to run"
        n197 = event-data() -> ("NewVal"=w323:u16)  [unwired: 1 in]
        n198 = property on="Test Name" class="Ring (strict)"() -> ("Strings []"=w324:string[])  [unwired: 2 in, 2 out]
        n199 = local write "Progress"(T7 {"Test Progress"=0, "Test Progress Text"=""} ("Progress")) -> ()
        n200 = Index Array(array=w324, index=w323) -> (element=w322:string)
        n201 = call <vilib>:"NT Write String.vi"("String"=w322, "Name"="/TestMode/TestName") -> ()  [unwired: 9 in, 1 out]
        n202 = property on="Progress" class="Clust (strict)"("Visible"=TRUE) -> ()  [unwired: 2 in, 2 out]
        n203 = property on="Motor" class="Clust (strict)"("Visible"=w319) -> ()  [unwired: 2 in, 2 out]
        n204 = property on="Test Slider" class="Slide (strict)"("Visible"=w319) -> ()  [unwired: 2 in, 2 out]
        n205 = property on="On/Off" class="Bool (strict)"("Visible"=w319) -> ()  [unwired: 2 in, 2 out]
        n206 = property on="Rev/Fwd" class="Clust (strict)"("Visible"=w319) -> ()  [unwired: 2 in, 2 out]
        n207 = property on="Test Ring" class="Ring (strict)"("Visible"=w319) -> ()  [unwired: 2 in, 2 out]
      }
      event "Select Auto": Mouse Enter {
        # "Populate the combo box with the list of autonomous options"
        n208 = event-data() -> ()  [unwired: 1 in, 1 out]
        n209 = call <vilib>:"NT Read String Array.vi"("Name"="Auto List") -> ("String Array"=w326:string[])  [unwired: 9 in, 1 out]
        n210 = property on="Select Auto" class="CmbBox"("Strings[]"=w326) -> ()  [unwired: 2 in, 2 out]
      }
      event "Select Auto": Value Change {
        # "User modified the Auto Selection. Write to NT variable so robot knows."
        n211 = event-data() -> ("NewVal"=w330:string)  [unwired: 1 in]
        n212 = call <vilib>:"NT Write String.vi"("String"=w330, "Name"="Auto Selector") -> ()  [unwired: 9 in, 1 out]
      }
      event "Command Selection": Value Change {
        # "Get the params and show in table"
        n213 = event-data() -> ("NewVal"=w337:i32)  [unwired: 1 in]
        n214 = property on="Command Selection" class="MCListbox (strict)"() -> ("ItemNames"=w335:string[][])  [unwired: 2 in, 2 out]
        n215 = call <vilib>:"WPI_DashboardUpdate Command Params.vi"("NewVal"=w337, "Commands"=w335, "Param Tbl"=w336) -> ()  [unwired: 8 in, 1 out]
      }
      event "Execute Command": Value Change {
        # "Started one, Unique ID holds\nresponse"
        n216 = event-data() -> ()  [unwired: 1 in, 1 out]
        n217 = property on="Command Selection" class="MCListbox (strict)"() -> ("ItemNames"=w349:string[][])  [unwired: 2 in, 2 out]
        n218 = Index Array(array=w349, index (row)="Command Selection", index (col)=0) -> (element=w347:string)
        n219 = call <vilib>:"Invoke Commands.vi"("Command Params"="Command Params", "Function Name"=w347) -> ("Params"=w343:u8, "Started"=w342:bool)  [unwired: 7 in, 1 out]
        n220 = Array Subset(array="Command Params", length (row)=w343) -> (w344:string[][])  [unwired: 3 in]
        n221 = Select(t="Executing" ("Cmd Status"), s=w342, f="" ("Cmd Status")) -> (s? t:f=→"Cmd Status":string)
      }
      event "Command Selection": Double Click {
        n222 = event-data() -> ("Row"=w359:i32)  [unwired: 1 in]
        n223 = property on="Command Selection" class="MCListbox (strict)"() -> ("ItemNames"=w362:string[][])  [unwired: 2 in, 2 out]
        n224 = local read "Command Params"() -> (w357:string[][])
        n225 = Index Array(array=w362, index (row)=w359, index (col)=0) -> (element=w360:string)
        n226 = call <vilib>:"Invoke Commands.vi"("Command Params"=w357, "Function Name"=w360) -> ("Params"=w356:u8, "Started"=w351:bool)  [unwired: 7 in, 1 out]
        n227 = Array Subset(array=w357, length (row)=w356) -> (w355:string[][])  [unwired: 3 in]
        n228 = Select(t="Executing" ("Cmd Status"), s=w351, f="" ("Cmd Status")) -> (s? t:f=w352:string)
        n229 = local write "Cmd Status"(w352) -> ()
      }
      event "CheckList": Double Click {
        # "Shift clears all"
        # "Update symbols on the listbox"
        n230 = event-data() -> ("PlatMods.Shift"=w365:bool, "Row"=w367:i32)  [unwired: 1 in]
        n231 = case shown="True" w365 {
          tunnel: w367 -> [w371 _]
          tunnel: 1 -> [w370 _]
          frame False {
            n232 = property on="CheckList" class="LstBox (strict)"() -> ("Item Symbols"=w369:i32[])  [unwired: 2 in, 2 out]
            n233 = Replace Array Subset(array=w369, new element=w370, index=w371) -> (w368:i32[])
            n234 = property on="CheckList" class="LstBox (strict)"("Item Symbols"=w368) -> ()  [unwired: 2 in, 2 out]
          }
          frame True {
            w372 = 0 ("Top Row")
            n235 = property on="CheckList" class="LstBox (strict)"() -> ("Number of Rows"=w374:u32)  [unwired: 2 in, 2 out]
            n236 = Initialize Array(0, w374) -> (w373:i32[])
            n237 = property on="CheckList" class="LstBox (strict)"("Top Row"=w372, "Value"=w372, "Item Symbols"=w373) -> ()  [unwired: 2 in, 2 out]
          }
        }
      }
      event "CheckList": Key Down {
        # "Update symbols on the listbox\nLeft and right keys check and uncheck"
        n238 = event-data() -> ("VKey"=w379:T22)  [unwired: 1 in]
        n239 = case shown="\"Left\", \"Right\"" w379 {
          selector: w379 -> [w384 _]
          tunnel: eventvkey."Left" ("VKey") -> [w382 _]
          frame "Left", "Right" {
            n240 = Equal?(x=w382, y=w384) -> (x = y?=w383:bool)
            n241 = Select(t=0, s=w383, f=1) -> (s? t:f=w385:i32)
            n242 = property on="CheckList" class="LstBox (strict)"() -> ("Item Symbols"=w388:i32[])  [unwired: 2 in, 2 out]
            n243 = Replace Array Subset(array=w388, new element=w385, index="CheckList") -> (w387:i32[])
            n244 = property on="CheckList" class="LstBox (strict)"("Item Symbols"=w387) -> ()  [unwired: 2 in, 2 out]
          }
          frame Default {
          }
        }
      }
      event "DB Camera Config": Value Change {
        # "Show or hide the cluster of controls, store in ini file"
        n245 = event-data() -> ("NewVal"=w393:bool)  [unwired: 1 in]
        n246 = case shown="False" w393 {
          tunnel: w392 -> [w402 _]
          tunnel: [w395 w413] -> w391
          tunnel: w390 -> [w394 w413]
          frame False {
            w409 = "Camera"
            w412 = FALSE ("Visible")
            n247 = local read "Camera Settings"() -> (w401:T2)
            n248 = Index Array(array=w402) -> (element=w405:cluster{string[]})  [unwired: 1 in]
            n249 = Unbundle(w401) -> ("Frame Rate"=w400:i32, "Compression"=w399:i32, "Size"=w403:u16)
            n250 = Unbundle(w405) -> (w404:string[])
            n251 = Index Array(array=w404, index=w403) -> (element=w398:string)
            n252 = call-poly <vilib>:"Write Key.vi"("section"=w409, "value"=w398, "key"="Size", "refnum"=w394) -> ("refnum out"=w411:T20)  [unwired: 2 in, 5 out]
            n253 = call-poly <vilib>:"Write Key.vi"("section"=w409, "value"=w400, "key"="FrameRate", "refnum"=w411) -> ("refnum out"=w410:T20)  [unwired: 1 in, 6 out]
            n254 = property on="Camera Settings" class="Clust (strict)"("Visible"=w412) -> ()  [unwired: 2 in, 2 out]
            n255 = local write "DB Camera Config"(w412) -> ()
            n256 = call-poly <vilib>:"Write Key.vi"("section"=w409, "value"=w399, "key"="Compression", "refnum"=w410) -> ("refnum out"=w396:T20)  [unwired: 1 in, 6 out]
            n257 = call <vilib>:"Close Config Data.vi"("refnum"=w396) -> ("file path"=w397:path)  [unwired: 2 in, 8 out]
            n258 = call <vilib>:"Open Config Data.vi"("configuration file path"=w397) -> ("refnum"=w395:T20)  [unwired: 8 in, 2 out]
          }
          frame True {
            n259 = property on="Camera Settings" class="Clust (strict)"("Visible"=TRUE) -> ()  [unwired: 2 in, 2 out]
          }
        }
      }
      event "Camera Settings": Value Change {
        # "Update summary string when any elements of DB camera change"
        n260 = event-data() -> ("NewVal"=w427:T2)  [unwired: 1 in]
        n261 = Index Array(array=w423) -> (element=w422:cluster{string[]})  [unwired: 1 in]
        n262 = Unbundle(w427) -> ("Frame Rate"=w418:i32, "Compression"=w417:i32, "Size"=w420:u16)
        n263 = Unbundle(w422) -> (w421:string[])
        n264 = Index Array(array=w421, index=w420) -> (element=w419:string)
        n265 = Format Into String(format string="%s   %dfps   %d%%", w419, w418, w417) -> (resulting string=w424:string)  [unwired: 2 in, 1 out]
        n266 = Build Array(w424) -> (w425:string[])
        n267 = property on="DB Camera Config" class="Bool (strict)"("Strings [4]"=w425) -> ()  [unwired: 2 in, 2 out]
      }
      event "Motor.Enable": Value Change {
        # "When the test mode otor enable helper is set, update that\ntree row item's value"
        n268 = event-data() -> ("NewVal"=w434:bool)  [unwired: 1 in]
        n269 = Unbundle("Motor") -> ("Value"=w433:dbl)  [unwired: 1 out]
        n270 = Select(t=w433, s=w434, f=0.0) -> (s? t:f=w431:dbl)
        n271 = call <vilib>:"NT Write Number.vi"("Numeric"=w431, "Name"=w430) -> ()  [unwired: 9 in, 1 out]
      }
      event "Test Slider": Value Change {
        # "When the test mode slider helper is set, update that\ntree row item's value"
        n272 = event-data() -> ("NewVal"=w438:dbl)  [unwired: 1 in]
        n273 = call <vilib>:"NT Write Number.vi"("Numeric"=w438, "Name"=w439) -> ()  [unwired: 9 in, 1 out]
      }
      event "On/Off": Value Change {
        # "When the test mode on/off helper value is set, update that\ntree row item's value"
        n274 = event-data() -> ("NewVal"=w444:bool)  [unwired: 1 in]
        n275 = Boolean To (0,1)(Boolean=w444) -> (0, 1=w443:i16)
        n276 = call <vilib>:"NT Write Number.vi"("Numeric"=w443, "Name"=w442) -> ()  [unwired: 9 in, 1 out]
      }
      event "Rev/Fwd": Value Change {
        # "When the test mode helper value for relays is set, update that\ntree row item's value"
        n277 = event-data() -> ("NewVal.Forward"=w453:bool, "NewVal.Reverse"=w452:bool)  [unwired: 1 in]
        n278 = Boolean To (0,1)(Boolean=w453) -> (0, 1=w449:i16)
        n279 = Boolean To (0,1)(Boolean=w452) -> (0, 1=w451:i16)
        n280 = Negate(x=w451) -> (-x=w450:i16)
        n281 = Add(x=w449, y=w450) -> (x+y=w448:i16)
        n282 = call <vilib>:"NT Write Number.vi"("Numeric"=w448, "Name"=w447) -> ()  [unwired: 9 in, 1 out]
      }
      event "Test Ring": Value Change {
        # "When a test mode helper value is selected from the ring,\nset the tree item's variable to the string value"
        n283 = event-data() -> ("NewVal"=w458:u16)  [unwired: 1 in]
        n284 = property on="Test Ring" class="Ring (strict)"() -> ("Strings []"=w459:string[])  [unwired: 2 in, 2 out]
        n285 = Index Array(array=w459, index=w458) -> (element=w457:string)
        n286 = call <vilib>:"NT Write String.vi"("String"=w457, "Name"=w456) -> ()  [unwired: 9 in, 1 out]
      }
      event "Rec Mode": Value Change {
        # "Update globals for recording mode and path to read log from.\nClear when logging and let NetworkTables set path for vision to\nuse."
        n287 = event-data() -> ("NewVal"=w471:enum32{"Stop", "Record", "Playback"})  [unwired: 1 in]
        n288 = global write "WPI_DashboardLogging Global.vi" "Logging Filename"(path "") -> ()
        n289 = global write "WPI_DashboardLogging Global.vi" "Recording"(w471) -> ()
        n290 = case shown="\"Playback\"" w471 {
          tunnel: w470 -> [_ w473 w482]
          tunnel: [_ _ w481] -> w467
          tunnel: [_ _ w480] -> _
          tunnel: w465 -> [_ _ w478]
          tunnel: cluster{i32, i32} {-250, 170} -> [_ _ w477]
          tunnel: [_ _ T23 {"Image Size"=TRUE, "Image Type"=TRUE, "Pixel Value"=TRUE, "ROI Information"=TRUE, "Zoom Factor"=FALSE} ("Image Information Shown:All Elements")] -> w463
          tunnel: [_ _ TRUE ("Zoom Factor")] -> w462
          tunnel: w461 -> [_ _ w474]
          frame Default {
          }
          frame "Stop", "Record" {
            # "Place Window too"
            n291 = invoke class="VI" method="FP.Close"(reference=w473) -> (reference out=w472:refnum<vi>)  [unwired: 2 in, 2 out]
            n292 = invoke class="VI" method="Abort VI"(reference=w472) -> ()  [unwired: 2 in, 3 out]
          }
          frame "Playback" {
            n293 = call "Open Playback Panel.vi"("Offset"=w477, "DB VI Ref"=w478, "Playback in"=w482) -> ("Playback out"=w479:refnum<vi>)  [unwired: 8 in]
            n294 = register-events(w479, w474) -> (reference out=w481:refnum<event-registration>, error out=w480:errorcluster)  [unwired: 2 in]
          }
        }
        n295 = property on="Camera Image" class="ImageControl"("Image Information Shown"=w463, "Image Information Visible"=w462) -> ()  [unwired: 2 in, 2 out]
        n296 = call <vilib>:"WPI_DashboardNT Log FieldName Cache.vi"("Operation"=enum16{"Lookup/Add", "Index", "Clear"}."Clear") -> ()  [unwired: 8 in, 3 out]
      }
      event Panel Close {
        w484 = enum32{"Stop", "Record", "Playback"}."Stop" ("Rec Mode")
        # "Playback window has been closed, abort"
        n297 = event-data() -> ()  [unwired: 1 in, 4 out]
        n298 = local write "Rec Mode"(w484) -> ()
        n299 = global write "WPI_DashboardLogging Global.vi" "Recording"(w484) -> ()
      }
      event Panel Close {
        # "Abort playback window and ourself"
        n300 = event-data() -> ()  [unwired: 1 in, 4 out]
        n301 = invoke class="VI" method="FP.Close"(reference=w490) -> (reference out=w489:refnum<vi>)  [unwired: 2 in, 2 out]
        n302 = invoke class="VI" method="Abort VI"(reference=w489) -> (error out=w488:errorcluster)  [unwired: 2 in, 2 out]
        n303 = invoke class="VI" method="Abort VI"(error in=w488) -> ()  [unwired: 2 in, 3 out]
      }
      event User Event {
        n304 = event-data() -> ("IDs"=w498:cluster{"RPC field ID":u16, "Unique ID":u16}, "String"=w497:string)  [unwired: 1 in]
        n305 = Bundle("IDs"=w498, "String"=w497) -> (w496:T9)  [unwired: 1 in]
        n306 = call <vilib>:"Retrieve RPC Response.vi"("RPC Response"=w496) -> ("Output"=w493:string[][])  [unwired: 10 in]
        n307 = Build Array (concatenate)(w491, w493) -> (w492:string[][])
        n308 = local write "Command Params"(w492) -> ()
        n309 = local write "Cmd Status"("" ("Cmd Status")) -> ()
      }
      event "Vision": Value Change {
        # "Enable/Disable Compression slider.\nHW USB is hard-coded into the camera"
        n310 = event-data() -> ("NewVal"=w505:u16)  [unwired: 1 in]
        n311 = Equal?(x=w505, y=u32 2 ("milliseconds to wait")) -> (x = y?=w503:bool)
        n312 = Select(t=T24."Disabled and Grayed Out" ("Disabled"), s=w503, f=T24."Enabled" ("Disabled")) -> (s? t:f=w500:T24)
        n313 = property on="Compression" class="Slide (strict)"("DisabledEnum"=w500) -> ()  [unwired: 2 in, 2 out]
      }
      event "Tree": Double Click {
        n314 = event-data() -> ("PlatMods"=w510:T27, "Tag"=w509:string)  [unwired: 1 in]
        n315 = Unbundle(w510) -> ("Shift"=w508:bool)  [unwired: 4 out]
        n316 = Not(x=w508) -> (.not. x?=w507:bool)
        n317 = call <vilib>:"NT Update Persistence.vi"("Persistence"=w507, "Name"=w509) -> ()  [unwired: 9 in, 1 out]
      }
    }
  }
  n318 = while {
    tunnel: w47 -> [w514]
    i -> [w517]
    stop <- FALSE stop-if-true
    n319 = Wait (ms)(milliseconds to wait=u32 100) -> ()  [unwired: 1 out]
    n320 = case shown="\"Playback\"" "Rec Mode" {
      tunnel: w517 -> [_ _ w532]
      tunnel: [u32 2829099 ("Base Color") u32 11141120 ("Target Color") w521] -> w513
      frame "Stop", Default {
        # "Reset the color, extra updates don't cost much"
      }
      frame "Record" {
      }
      frame "Playback" {
        # "Playback"
        n321 = Quotient & Remainder(x=w532, y=u32 50 ("milliseconds to wait")) -> (x-y*floor(x/y)=w528:u32)  [unwired: 1 out]
        n322 = Divide(x=w528, y=u32 50 ("milliseconds to wait")) -> (x/y=w525:dbl)
        n323 = Multiply(x=6.283185307179586, y=w525) -> (x*y=w530:dbl)
        n324 = Sine(x=w530) -> (sin(x)=w529:dbl)
        n325 = Absolute Value(x=w529) -> (abs(x)=w522:dbl)
        n326 = call "Interpolate RGB Color.vi"("Proportion"=w522, "Target Color"=u32 30976, "Base Color"=u32 2829099) -> ("Result Color"=w521:u32)  [unwired: 8 in]
      }
    }
    n327 = property class="Pane"(reference=w514, "PaneColor"=w513) -> ()  [unwired: 1 in, 2 out]
  }
  n328 = local write "Dashboard Tab"(T1."Drive" ("Dashboard Tab")) -> ()
  n329 = property on="On/Off" class="Bool (strict)"("Visible"=w15) -> ()  [unwired: 2 in, 2 out]
  n330 = property on="Motor" class="Clust (strict)"("Visible"=w15) -> ()  [unwired: 2 in, 2 out]
  n331 = property on="Progress" class="Clust (strict)"("Visible"=w15) -> ()  [unwired: 2 in, 2 out]
  n332 = property on="Test Ring" class="Ring (strict)"("Visible"=w15) -> ()  [unwired: 2 in, 2 out]
  n333 = property on="Rev/Fwd" class="Clust (strict)"("Visible"=w15) -> ()  [unwired: 2 in, 2 out]
  n334 = property on="Camera Settings" class="Clust (strict)"("Visible"=w15) -> ()  [unwired: 2 in, 2 out]
  n335 = while {
    tunnel: u16 1741 ("timeout ms (25000)") -> [w534]
    stop <- FALSE stop-if-true
    n336 = TCP Create Listener(10:w534) -> (0:w533:errorcluster, 3:w535:refnum<k5>)  [unwired: 4 in, 1 out]
    n337 = case shown="No Error" w533 {
      selector: w533 -> [w537 _]
      tunnel: w535 -> [w538 _]
      frame No Error {
        n338 = while {
          tunnel: w538 -> [w541]
          tunnel: w537 -> [w540]
          stop <- FALSE stop-if-true
          n339 = TCP Wait On Listener(8:w540, 11:w541) -> (0:w542:errorcluster, 4:w543:refnum<k5>)  [unwired: 2 in, 3 out]
          n340 = local write "TCP"(w543) -> ()
          n341 = case shown="No Error" w542 {
            frame No Error {
            }
            frame Error {
              n342 = Wait (ms)(milliseconds to wait=u32 1000) -> ()  [unwired: 1 out]
            }
          }
        }
      }
      frame Error {
        n343 = Wait (ms)(milliseconds to wait=u32 1000) -> ()  [unwired: 1 out]
      }
    }
  }
  n344 = local write "DB Camera Config"(w15) -> ()
  n345 = local write "Command Params"(string[][] [] ("Command Params")) -> ()
  n346 = global write "WPI_DashboardLogging Global.vi" "Recording"(w41) -> ()
  n347 = local write "Command Selection"(u16 0 ("milliseconds to wait")) -> ()
  n348 = local write "Rec Mode"(w41) -> ()
